vi "Stop_Meas_Prog.vi"() -> (5 "Plug in titles":string[](array[string]), 7 "Plug in values":string[](array[string]))   [LabVIEW 2020]
uses:
  Globals/Trav_pos_global.vi
  Globals/Meas_global.vi
panel:
  in  "Stop Button":bool
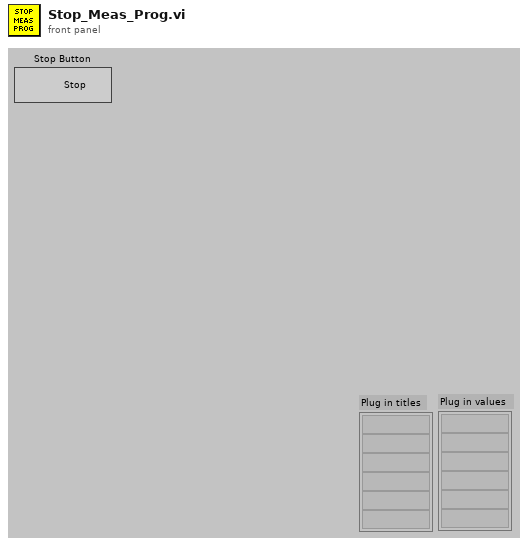
[diagram p1: front panel]
types:
  T1 = typedef "Post_Process.ctl" = enum16{"Take New Data", "Post Process Raw Data File"}
  T2 = enum32{"Bad", "Idle", "Run top level", "Running"}
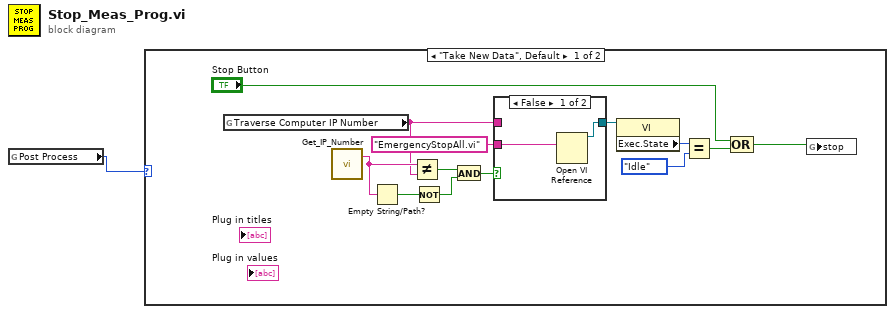
[diagram p0: block diagram]
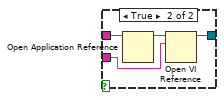
[diagram p2: hidden frame]
diagram:
  n1 = global read "Meas_global.vi" "Post Process"() -> (w1:T1)
  n2 = case shown="\"Take New Data\", Default" w1 {
    frame "Take New Data", Default {
      n3 = global read "Trav_pos_global.vi" "Traverse Computer IP Number"() -> (w6:string)
      n4 = call "Get_IP_Number.vi"() -> ("IP Number"=w11:string)  [unwired: 1 out]
      n5 = Empty String/Path?(string/path=w11) -> (empty?=w8:bool)
      n6 = Not Equal?(x=w11, y=w6) -> (x != y?=w10:bool)
      n7 = Not(x=w8) -> (.not. x?=w9:bool)
      n8 = And(x=w10, y=w9) -> (x .and. y?=w7:bool)
      n9 = case shown="False" w7 {
        tunnel: [w16 w19] -> w5
        tunnel: w6 -> [_ w20]
        tunnel: "EmergencyStopAll.vi" -> [w15 w17]
        frame False {
          n10 = Open VI Reference(vi path=w15) -> (vi reference=w16:refnum<vi>)  [unwired: 5 in, 1 out]
        }
        frame True {
          n11 = Open Application Reference(11:w20) -> (3:w18:refnum<vi>)  [unwired: 2 in, 2 out]
          n12 = Open VI Reference(application reference (local)=w18, vi path=w17) -> (vi reference=w19:refnum<vi>)  [unwired: 4 in, 1 out]
        }
      }
      n13 = property class="VI"(reference=w5) -> ("Exec.State"=w13:T2)  [unwired: 1 in, 2 out]
      n14 = Equal?(x=w13, y=T2."Idle") -> (x = y?=w3:bool)
      n15 = Compound Arithmetic op=OR("Stop Button", w3) -> (w2:bool)
      n16 = global write "Meas_global.vi" "stop"(w2) -> ()
    }
    frame "Post Process Raw Data File" {
    }
  }
